vi "INTRO.vi"(10 "Boolean 2":refnum<vi>) -> ()   [LabVIEW 2019]
panel:
  out "Slide":u8(slide) scale=0.0..100.0
  # "PUMPTEST 2023"
  # "AVVIO IN CORSO ........"
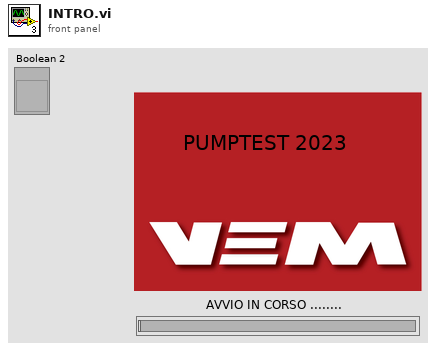
[diagram p1: front panel]
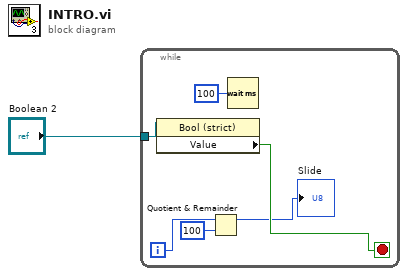
[diagram p0: block diagram]
diagram:
  n1 = while {
    tunnel: "Boolean 2" -> [w6]
    i -> [w4]
    stop <- w5 stop-if-true
    n2 = property class="Bool (strict)"(reference=w6) -> ("Value"=w5:bool)  [unwired: 1 in, 2 out]
    n3 = Quotient & Remainder(x=w4, y=100) -> (x-y*floor(x/y)=→"Slide":i32)  [unwired: 1 out]
    n4 = Wait (ms)(milliseconds to wait=u32 100) -> ()  [unwired: 1 out]
  }
